vi "current_vrs_time_cluster.vi"(0 "Input data":dbl[][](array[numeric]), 1 "Clear Graph?":bool, 2 "Time":dbl, 4 "?":T1=enum."VCC", 5 "sensitivity (V/A)":dbl, 6 "VCC":dbl) -> (7 "rms value":dbl format="%0.2f", 8 "Cluster":cluster{dbl[], dbl[]})   [LabVIEW 2016]
uses:
  INPUTS.ctl
  <vilib>/Analysis/5stat.llb/RMS (DBL).vi
  <vilib>/Analysis/NI_AALPro.lvlib
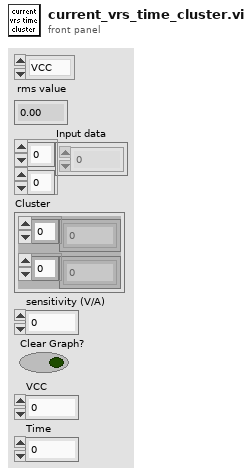
[diagram p1: front panel]
types:
  T1 = typedef "INPUTS.ctl" = enum16{"I_CELL", "I_LOAD", "I_PV", "V_BUS", "V_CELL", "VCC"}
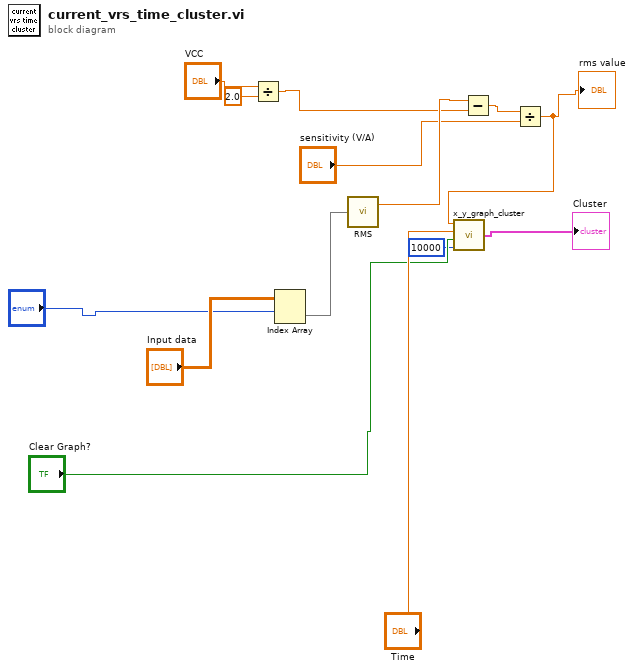
[diagram p0: block diagram]
diagram:
  n1 = Divide(x="VCC", y=2.0) -> (x/y=w4:dbl)
  n2 = Index Array(array="Input data", index (row)="?") -> (element=w14:dbl[])  [unwired: 1 in]
  n3 = call-poly <vilib>:"RMS.vi"("X"=w14) -> ("rms value"=w5:dbl)  [unwired: 1 out]
  n4 = Subtract(x=w5, y=w4) -> (x-y=w3:dbl)
  n5 = Divide(x=w3, y="sensitivity (V/A)") -> (x/y=w1:dbl)
  "rms value" <- w1
  n6 = call "x_y_graph_cluster.vi"("Chart History (10,000)"=10000, "Clear Graph?"="Clear Graph?", "X"="Time", "Y"=w1) -> ("Cluster"=→"Cluster":cluster{dbl[], dbl[]})
